vi "APPLY NEXT TEMP.vi"(6 "Numeric in":i32, 7 "Field and Temp Range":T1={"VISA (Magnet)"="COM4", "Fields(T)"=[], "Temps(K)"=[], "VISA (Temp) "="COM1"}, 8 "error in (no error)":errorcluster, 9 "element in":T2 {"Output's Control Loop (1:1)" items=["1"=1, "2"=2]; "Data Source (0:Kelvin)" items=["Kelvin", "Celsius", "Sensor Units"]; "Input (0:A)" items=["A", "B", "C", "D", "D2", "D3", "D4", "D5"]; "Configure Control Parameters (0: Configure)" items=["Configure", "Don't Configure"]; "Serial Configuration"."Flow Control" items=["None", "XON/XOFF", "RTS/CTS", "XON/XOFF & RTS/CTS", "DTR/DSR", "XON/XOFF & DTR/DSR"]; "Serial Configuration"."Stop Bits" items=["1.0"=10, "1.5"=15, "2.0"=20]; "Serial Configuration"."Data Bits" items=["7"=7, "8"=8]; "Serial Configuration"."Parity" items=["None", "Odd", "Even", "Mark", "Space"]; "Serial Configuration"."Baud Rate" items=["300"=300, "600"=600, "1200"=1200, "2400"=2400, "4800"=4800, "9600"=9600, "19200"=19200, "38400"=38400, "57600"=57600]; "Target Temp (K)" format="%.5f"; "Input (0:None)" items=["None", "A", "B", "C", "D", "D2", "D3", "D4", "D5"]; "Mode (0:Off)" items=["Off", "Closed Loop PID", "Zone", "Open Loop"]; "Heater Out Display (1:Current)" items=["Current"=1, "Power"=2]; "Max Current (0:User Specified)" items=["User Specified", "0.707 A", "1.0 A", "1.141 A", "2.0 A"]; "Heater Resistance (1:25 Ohms)" items=["25 Ohms"=1, "50 Ohms"=2]; "Max User Current (2.000)" format="%.3f"; "Gain (P) (50.0)" format="%.1f"; "Reset (I) (20.0)" format="%.1f"; "Rate (D) (0.0 %)" format="%.1f"; "Manual Output (0.00 %)" format="%.2f"; "Range (0:Off)" items=["Off", "Range 1 (On)", "Range 2", "Range 3", "Range 4", "Range 5"]}, 10 "TempQ in":refnum<queue>, 11 "VISA Refnum in":refnum<visa-resource-name>) -> (0 "error out":errorcluster, 1 "Numeric out":i32, 2 "TempQ out":refnum<queue>, 3 "VISA Refnum out":refnum<visa-resource-name>, 5 "New SP":dbl)   [LabVIEW 2025]
uses:
  Temp Cntrl.ctl
  <instrlib>/Lake Shore 350/Lake Shore 350.lvlib
  <userlib>/Nanonis Prog Interface V5e/Nanonis Prog Interface.lvlib
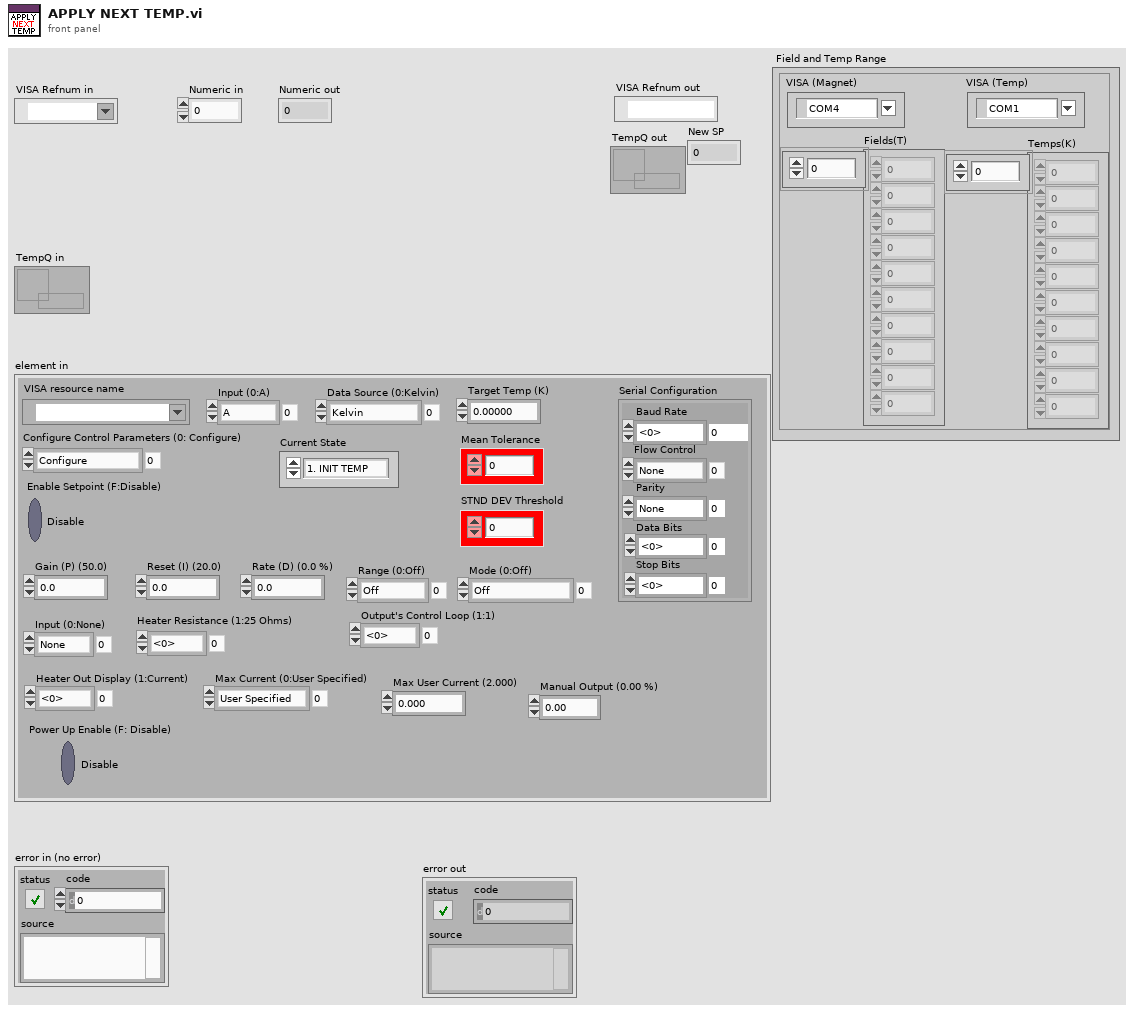
[diagram p1: front panel]
types:
  T1 = cluster{"VISA (Magnet)":refnum<visa-resource-name>, "Fields(T)":dbl[], "Temps(K)":dbl[], "VISA (Temp) ":refnum<visa-resource-name>}
  T2 = typedef "Temp Cntrl.ctl" = cluster{"Range (0:Off)":u16, "Manual Output (0.00 %)":dbl, "Rate (D) (0.0 %)":dbl, "Reset (I) (20.0)":dbl, "Gain (P) (50.0)":dbl, "Power Up Enable (F: Disable)":bool, "Max User Current (2.000)":dbl, "Heater Resistance (1:25 Ohms)":u16, "Max Current (0:User Specified)":u16, "Heater Out Display (1:Current)":u16, "Mode (0:Off)":u16, "Input (0:None)":u16, "Target Temp (K)":dbl, "Serial Configuration":cluster{"Baud Rate":u32, "Parity":u16, "Data Bits":u16, "Stop Bits":u16, "Flow Control":u16}, "VISA resource name":refnum<visa-resource-name>, "Configure Control Parameters (0: Configure)":u16, "Enable Setpoint (F:Disable)":bool, "Input (0:A)":u16, "Data Source (0:Kelvin)":u16, "Output's Control Loop (1:1)":u16, "STND DEV Threshold ":dbl, "Mean Tolerance ":dbl, "Current State":enum16{"1. INIT TEMP", "2. TC ON", "3. POLL_TEMPS", "4. TEMP_STAB", "5. TC IDLE", "6. APPLY NEXT TEMP", "7. TC OFF (Reset)"}}
  T3 = enum16{"1. INIT TEMP", "2. TC ON", "3. POLL_TEMPS", "4. TEMP_STAB", "5. TC IDLE", "6. APPLY NEXT TEMP", "7. TC OFF (Reset)"}
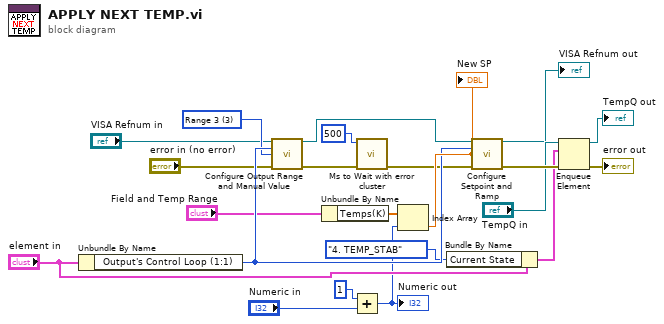
[diagram p0: block diagram]
diagram:
  w12 = u16 3 items=["Off", "Range 1 (On)", "Range 2", "Range 3", "Range 4", "Range 5"] ("Range (0:Off)")
  n1 = Unbundle By Name("element in") -> ("Output's Control Loop (1:1)"=w14:u16)
  n2 = call <instrlib>:"Configure Output Range and Manual Value.vi"("VISA resource name"="VISA Refnum in", "Output (1:1)"=w14, "Range (0:Off)"=w12, "error in (no error)"="error in (no error)") -> ("VISA resource name out"=w13:refnum<visa-resource-name>, "error out"=w2:errorcluster)  [unwired: 10 in]
  n3 = Unbundle By Name("Field and Temp Range") -> ("Temps(K)"=w6:dbl[])
  n4 = Add(x=1, y="Numeric in") -> (x+y=w9:i32)
  "Numeric out" <- w9
  n5 = call <userlib>:"Ms to Wait with error cluster.vi"("error in (no error)"=w2, "milliseconds to wait"=u32 500) -> ("error out"=w1:errorcluster)  [unwired: 4 in, 1 out]
  n6 = Index Array(array=w6, index=w9) -> (element=w15:dbl)
  "New SP" <- w15
  n7 = Bundle By Name(cluster="element in", "Current State"=T3."4. TEMP_STAB") -> (w19:T2)
  n8 = call <instrlib>:"Configure Setpoint and Ramp.vi"("VISA resource name"=w13, "Output's Control Loop (1:1)"=w14, "Setpoint (0.00000)"=w15, "error in (no error)"=w1) -> ("VISA resource name out"=→"VISA Refnum out":refnum<visa-resource-name>, "error out"=w21:errorcluster)  [unwired: 10 in]
  n9 = Enqueue Element(queue="TempQ in", element=w19, error in (no error)=w21) -> (queue out=→"TempQ out":refnum<queue>, error out=→"error out":errorcluster)  [unwired: 1 in, 1 out]
